vi "Create_and_save_to_file (SubVI).vi"(2 "input string":string, 3 "error in":errorcluster) -> (6 "Текущее расположение файла":path, 7 "error out":errorcluster)   [LabVIEW 2015]
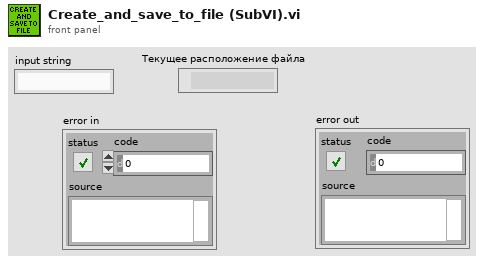
[diagram p1: front panel]
types:
  T1 = enum16{"open", "replace", "create", "open or create", "replace or create", "replace or create with confirmation"}
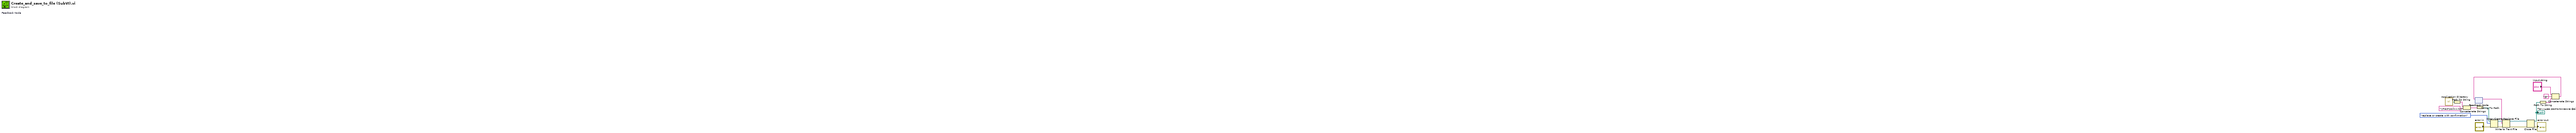
[diagram p0: block diagram]
diagram:
  n1 = call <vilib>:"Application Directory.vi"() -> ("Application Directory"=w6:path)
  n2 = Path To String(path=w6) -> (string=w5:string)
  n3 = Concatenate Strings(w5, "\\Настройки.txt" ("prompt (Open existing file)")) -> (w4:string)
  n4 = feedback #1 "Feedback Node"() -> (w9:string)  [unwired: 1 in]
  n5 = String To Path(string=w4) -> (path=w1:path)
  n6 = Open/Create/Replace File(file path (use dialog)=w1, error in="error in", operation (0:open)=T1."replace or create with confirmation") -> (refnum out=w16:refnum<file>, error out=w18:errorcluster)  [unwired: 4 out]
  n7 = Write to Text File(file (use dialog)=w16, text=w9, error in=w18) -> (refnum out=w13:refnum<file>, error out=w15:errorcluster)  [unwired: 2 out]
  n8 = Close File(refnum=w13, error in=w15) -> (path=w12:path, error out=→"error out":errorcluster)
  "Текущее расположение файла" <- w12
  n9 = Path To String(path=w12) -> (string=w7:string)
  n10 = Concatenate Strings("input string", "@" ("string"), w7) -> (w10:string)
  n11 = feedback-in #1(w10) -> ()
